vi "Control-GetContrast.vi"(5 "Streeam?":bool, 6 "Image Device IN":cluster{"Image":T2, "errorImage":errorcluster}, 7 "Camera Device  IN":T1) -> (1 "Contraste OUT":dbl, 2 "Image Device OUT":cluster{"Image":T2, "errorImage":errorcluster}, 3 "Camera Device OUT":T1)   [LabVIEW 2010]
uses:
  <vilib>/vision/Image Controls.llb/IMAQ Image.ctl
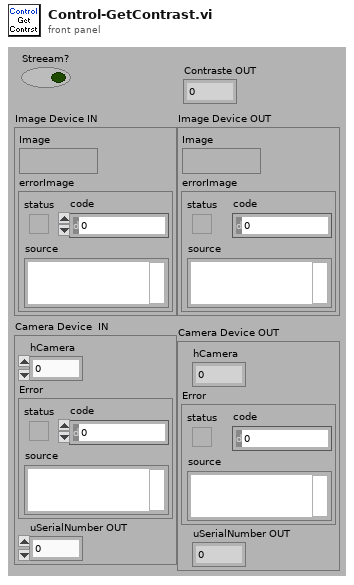
[diagram p1: front panel]
types:
  T1 = cluster{"hCamera":u32, "Error":errorcluster, "uSerialNumber OUT":u32}
  T2 = typedef "IMAQ Image.ctl" = refnum<image>
  T3 = cluster{"hCamera":u32, "Error":errorcluster, "uSerialNumber":u32}
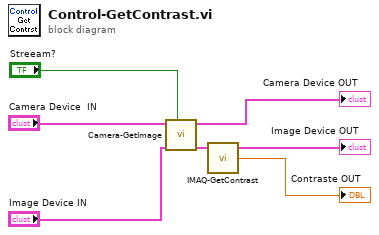
[diagram p0: block diagram]
diagram:
  n1 = call "Camera-GetImage.vi"("Streeam"="Streeam?", "Image Device IN"="Image Device IN", "Camera Device IN"="Camera Device  IN") -> ("Image Device OUT"=w3:cluster{"Image":T2, "errorImage":errorcluster}, "Camera Device OUT"=→"Camera Device OUT":T3)  [unwired: 4 in]
  n2 = call "IMAQ-GetContrast.vi"("Image Device IN"=w3) -> ("RMS Contraste"=→"Contraste OUT":dbl, "Image Device OUT"=→"Image Device OUT":cluster{"Image":T2, "errorImage":errorcluster})  [unwired: 3 in]
